vi "TestSurface.vi"() -> ()   [LabVIEW 2024]
uses:
  SDL3/Init/InitFlags--ring.ctl
  <vilib>/picture/picture.llb/imagedata.ctl
  SDL3/Pixels/PixelFormat--enum.ctl
  SDL3/Rect/Rect--cluster.ctl
  SDL3/Init/Init.lvlib
  SDL3/Surface/Surface.lvlib
  SDL3/Rect/Rect.lvlib
  SDL3/Pixels/Pixels.lvlib
  SDL3/Video/Video.lvlib
  SDL3/Video/WindowFlags--ring.ctl
  SDL3/Render/Render.lvlib
  SDL3/Render/TextureAccess-enum.ctl
panel:
  out "new picture 2":picture
  out "color":u32=16711680 format="%06x"
  out "new picture":picture
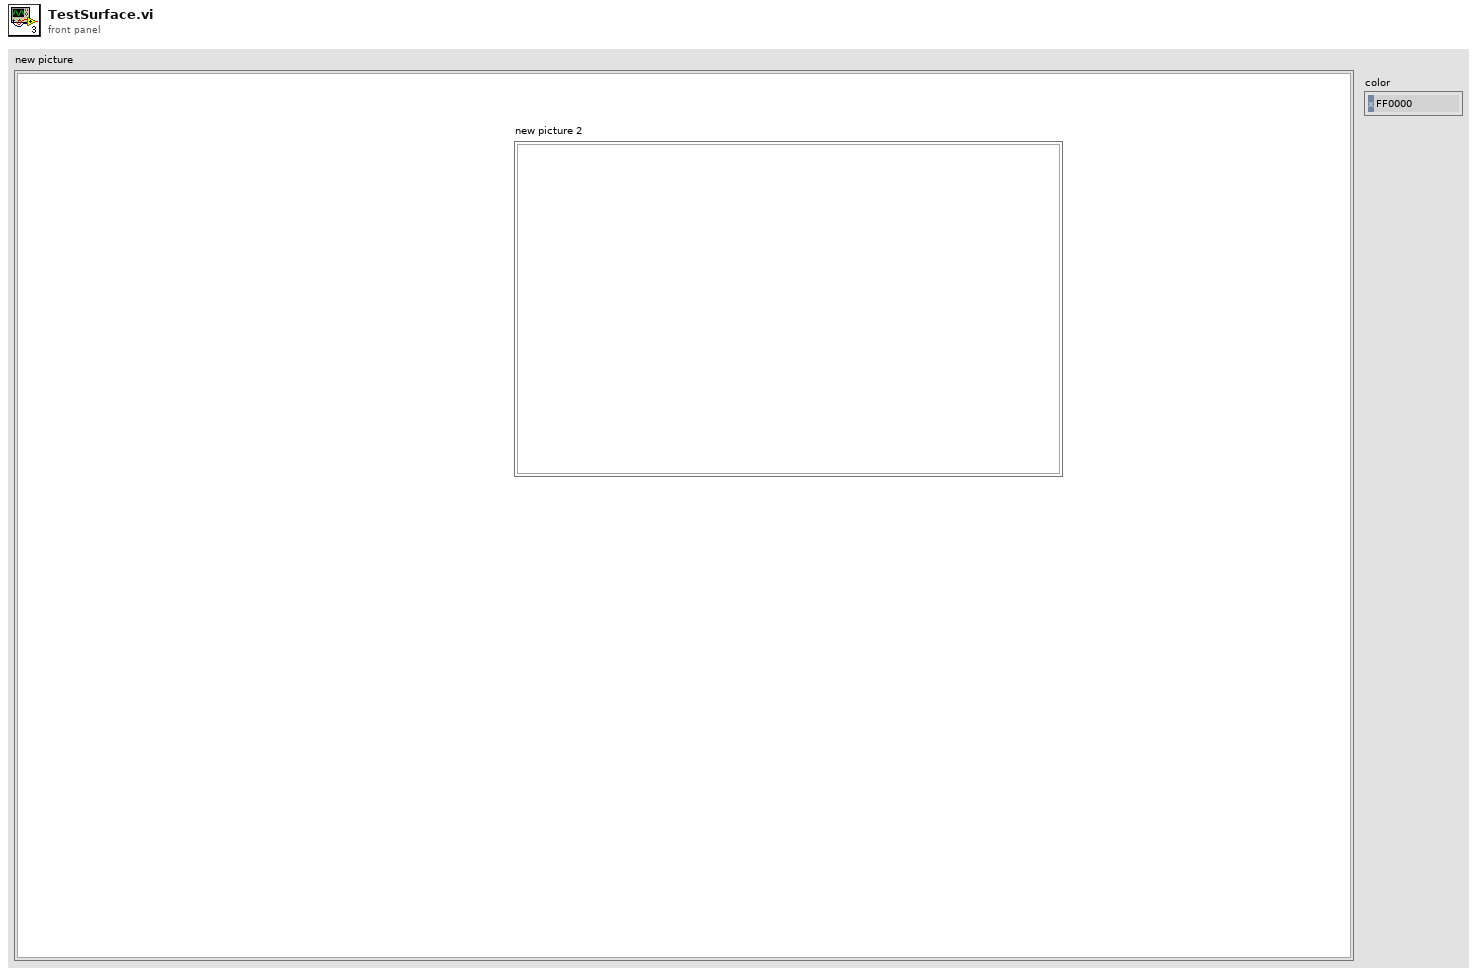
[diagram p1: front panel]
types:
  T1 = typedef "imagedata.ctl" = cluster{"image type":i32, "image depth":i32, "image":u8[], "mask":u8[], "colors":u32[], "Rectangle":cluster{"left":i16, "top":i16, "right":i16, "bottom":i16}}
  T2 = cluster{"left":i16, "top":i16, "right":i16, "bottom":i16}
  T3 = typedef "SDL3.lvlib/Init.lvlib/InitFlags--ring.ctl" = u32
  T4 = typedef "SDL3.lvlib/Render.lvlib/TextureAccess-enum.ctl" = enum32{"SDL_TEXTUREACCESS_STATIC", "SDL_TEXTUREACCESS_STREAMING", "SDL_TEXTUREACCESS_TARGET"}
  T5 = typedef "SDL3.lvlib/Pixels.lvlib/PixelFormat--enum.ctl" = enum32{"SDL_PIXELFORMAT_UNKNOWN", "SDL_PIXELFORMAT_INDEX1LSB", "SDL_PIXELFORMAT_INDEX1MSB", "SDL_PIXELFORMAT_INDEX2LSB", "SDL_PIXELFORMAT_INDEX2MSB", "SDL_PIXELFORMAT_INDEX4LSB", "SDL_PIXELFORMAT_INDEX4MSB", "SDL_PIXELFORMAT_INDEX8", "SDL_PIXELFORMAT_RGB332", "SDL_PIXELFORMAT_XRGB4444", "SDL_PIXELFORMAT_XBGR4444", "SDL_PIXELFORMAT_XRGB1555", "SDL_PIXELFORMAT_XBGR1555", "SDL_PIXELFORMAT_ARGB4444", "SDL_PIXELFORMAT_RGBA4444", "SDL_PIXELFORMAT_ABGR4444", "SDL_PIXELFORMAT_BGRA4444", "SDL_PIXELFORMAT_ARGB1555", "SDL_PIXELFORMAT_RGBA5551", "SDL_PIXELFORMAT_ABGR1555", "SDL_PIXELFORMAT_BGRA5551", "SDL_PIXELFORMAT_RGB565", "SDL_PIXELFORMAT_BGR565", "SDL_PIXELFORMAT_RGB24", "SDL_PIXELFORMAT_BGR24", "SDL_PIXELFORMAT_XRGB8888", "SDL_PIXELFORMAT_RGBX8888", "SDL_PIXELFORMAT_XBGR8888", "SDL_PIXELFORMAT_BGRX8888", "SDL_PIXELFORMAT_ARGB8888", "SDL_PIXELFORMAT_RGBA8888", "SDL_PIXELFORMAT_ABGR8888", "SDL_PIXELFORMAT_BGRA8888", "SDL_PIXELFORMAT_XRGB2101010", "SDL_PIXELFORMAT_XBGR2101010", "SDL_PIXELFORMAT_ARGB2101010", "SDL_PIXELFORMAT_ABGR2101010", "SDL_PIXELFORMAT_RGB48", "SDL_PIXELFORMAT_BGR48", "SDL_PIXELFORMAT_RGBA64", "SDL_PIXELFORMAT_ARGB64", "SDL_PIXELFORMAT_BGRA64", "SDL_PIXELFORMAT_ABGR64", "SDL_PIXELFORMAT_RGB48_FLOAT", "SDL_PIXELFORMAT_BGR48_FLOAT", "SDL_PIXELFORMAT_RGBA64_FLOAT", "SDL_PIXELFORMAT_ARGB64_FLOAT", "SDL_PIXELFORMAT_BGRA64_FLOAT", "SDL_PIXELFORMAT_ABGR64_FLOAT", "SDL_PIXELFORMAT_RGB96_FLOAT", "SDL_PIXELFORMAT_BGR96_FLOAT", "SDL_PIXELFORMAT_RGBA128_FLOAT", "SDL_PIXELFORMAT_ARGB128_FLOAT", "SDL_PIXELFORMAT_BGRA128_FLOAT", "SDL_PIXELFORMAT_ABGR128_FLOAT", "SDL_PIXELFORMAT_YV12", "SDL_PIXELFORMAT_IYUV", "SDL_PIXELFORMAT_YUY2", "SDL_PIXELFORMAT_UYVY", "SDL_PIXELFORMAT_YVYU", "SDL_PIXELFORMAT_NV12", "SDL_PIXELFORMAT_NV21", "SDL_PIXELFORMAT_P010", "SDL_PIXELFORMAT_EXTERNAL_OES"}
  T6 = typedef "SDL3.lvlib/Video.lvlib/WindowFlags--ring.ctl" = u64
  T7 = typedef "SDL3.lvlib/Rect.lvlib/Rect--cluster.ctl" = cluster{"x":i32, "y":i32, "w":i32, "h":i32}
  T8 = typedef "SDL3.lvlib/Surface.lvlib/SurfaceFlags--ring.ctl" = u32
  T9 = cluster{"flag":T8, "format":T5, "w":i32, "h":i32, "pitch":i32}
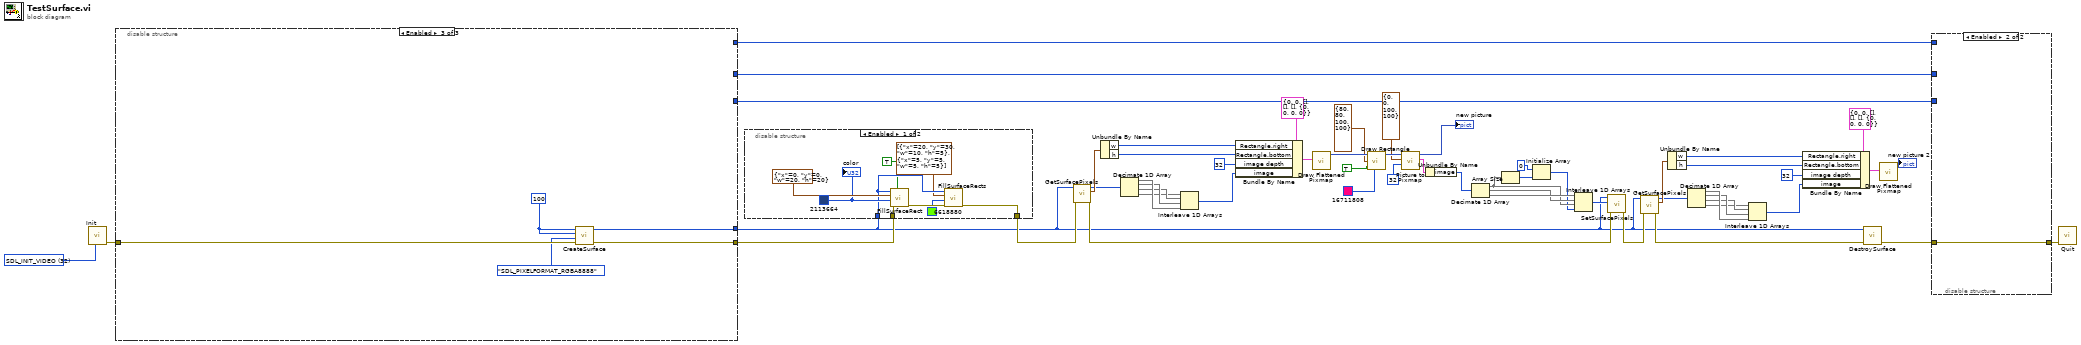
[diagram p0: block diagram]
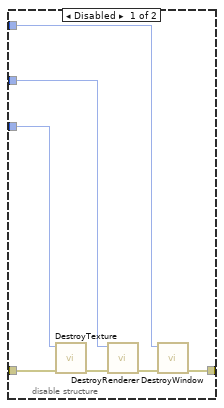
[diagram p2: hidden frame]
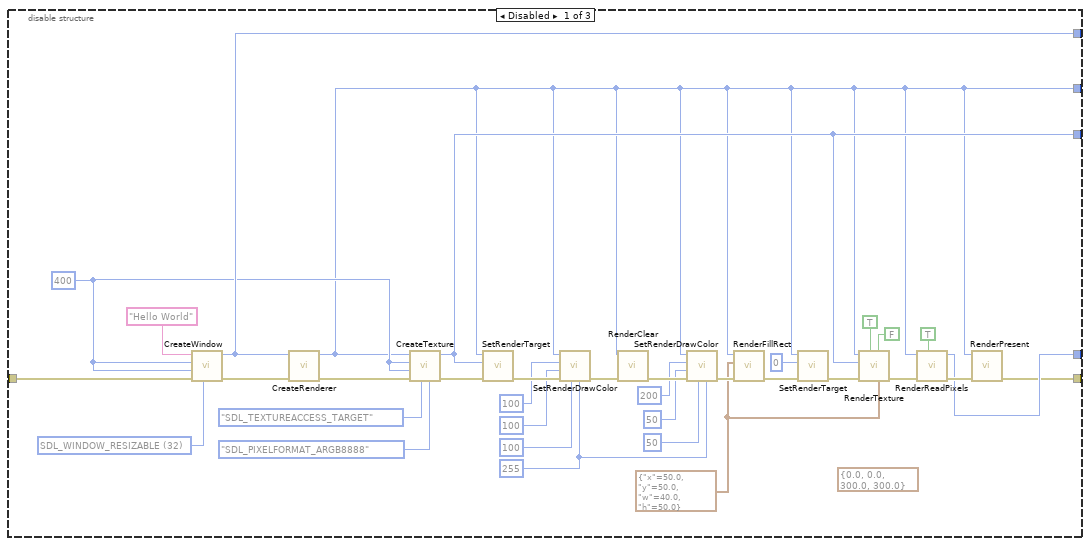
[diagram p3: hidden frame]
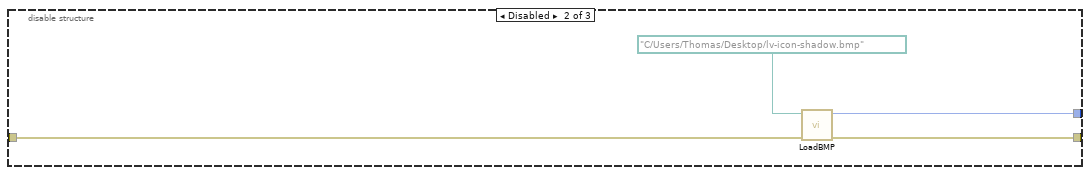
[diagram p4: hidden frame]
diagram:
  w55 = T3 32 items=["NONE"=0, "SDL_INIT_AUDIO"=16, "SDL_INIT_VIDEO"=32, "SDL_INIT_JOYSTICK"=512, "SDL_INIT_HAPTIC"=4096, "SDL_INIT_GAMEPAD"=8192, "SDL_INIT_EVENTS"=16384, "SDL_INIT_SENSOR"=32768, "SDL_INIT_CAMER"=65536] ("InitFlags")
  n1 = call "Init.vi"("InitFlags"=w55) -> ("error out"=w53:errorcluster)  [unwired: 10 in]
  n2 = disable-structure shown="Enabled" {
    disable-tunnel: w53 -> [w84 w93 w98]
    disable-tunnel: [w65 _ _] -> w50
    disable-tunnel: [w64 _ _] -> w49
    disable-tunnel: [w59 w91 w95] -> w1
    disable-tunnel: [w58 w92 w97] -> w47
    disable-tunnel: [w56 _ _] -> w46
    frame Disabled {
      w63 = cluster{"x":sgl, "y":sgl, "w":sgl, "h":sgl} {"x"=50.0, "y"=50.0, "w"=40.0, "h"=50.0} ("rect")
      w68 = u8 255 ("a")
      (unwired) cluster{"x":sgl, "y":sgl, "w":sgl, "h":sgl} {"x"=0.0, "y"=0.0, "w"=300.0, "h"=300.0} ("dstrect")
      w62 = 400 ("h")
      w88 = T6 32 items=["0"=0, "SDL_WINDOW_FULLSCREEN"=1, "SDL_WINDOW_OPENGL"=2, "SDL_WINDOW_OCCLUDED"=4, "SDL_WINDOW_HIDDEN"=8, "SDL_WINDOW_BORDERLESS"=16, "SDL_WINDOW_RESIZABLE"=32, "SDL_WINDOW_MINIMIZED"=64, "SDL_WINDOW_MAXIMIZED"=128, "SDL_WINDOW_MOUSE_GRABBED"=256, "SDL_WINDOW_INPUT_FOCUS"=512, "SDL_WINDOW_MOUSE_FOCUS"=1024, "SDL_WINDOW_EXTERNAL"=2048, "SDL_WINDOW_MODAL"=4096, "SDL_WINDOW_HIGH_PIXEL_DENSITY"=8192, "SDL_WINDOW_MOUSE_CAPTURE"=16384, "SDL_WINDOW_MOUSE_RELATIVE_MODE"=32768, "SDL_WINDOW_ALWAYS_ON_TOP"=65536, "SDL_WINDOW_UTILITY"=131072, "SDL_WINDOW_TOOLTIP"=262144, "SDL_WINDOW_POPUP_MENU"=524288, "SDL_WINDOW_KEYBOARD_GRABBED"=1048576, "SDL_WINDOW_VULKAN"=268435456, "SDL_WINDOW_METAL"=536870912, "SDL_WINDOW_TRANSPARENT"=1073741824, "SDL_WINDOW_NOT_FOCUSABLE"=2147483648] ("flags (0)")
      n3 = call "CreateWindow.vi"("flags (0)"=w88, "No Error"=w84, "h"=w62, "w"=w62, "title"="Hello World") -> ("error out"=w87:errorcluster, "window [SDL_Window *]"=w64:i64)  [unwired: 5 in]
      n4 = call "CreateRenderer.vi"("No Error"=w87, "window [SDL_Window *]"=w64) -> ("error out"=w86:errorcluster, "renderer [SDL_Renderer *]"=w56:i64)  [unwired: 8 in]
      n5 = call "CreateTexture.vi"("pixel_format"=PixelFormat--enum."SDL_PIXELFORMAT_ARGB8888", "texture_access"=TextureAccess-enum."SDL_TEXTUREACCESS_TARGET", "No Error"=w86, "h"=w62, "w"=w62, "renderer [SDL_Renderer *]"=w56) -> ("error out"=w66:errorcluster, "texture [SDL_Texture *]"=w65:i64)  [unwired: 4 in]
      n6 = call "SetRenderTarget.vi"("No Error"=w66, "texture [SDL_Texture *]"=w65, "renderer [SDL_Renderer *]"=w56) -> ("error out"=w81:errorcluster)  [unwired: 8 in]
      n7 = call "SetRenderDrawColor.vi"("a"=w68, "b"=u8 100, "No Error"=w81, "g"=u8 100, "r"=u8 100, "renderer [SDL_Renderer *]"=w56) -> ("error out"=w79:errorcluster)  [unwired: 5 in]
      n8 = call "RenderClear.vi"("No Error"=w79, "renderer [SDL_Renderer *]"=w56) -> ("error out"=w80:errorcluster)  [unwired: 9 in]
      n9 = call "SetRenderDrawColor.vi"("a"=w68, "b"=u8 50, "No Error"=w80, "g"=u8 50, "r"=u8 200, "renderer [SDL_Renderer *]"=w56) -> ("error out"=w72:errorcluster)  [unwired: 5 in]
      n10 = call "RenderFillRect.vi"("No Error"=w72, "rect"=w63, "renderer [SDL_Renderer *]"=w56) -> ("error out"=w67:errorcluster)  [unwired: 8 in]
      n11 = call "SetRenderTarget.vi"("No Error"=w67, "texture [SDL_Texture *]"=i64 0, "renderer [SDL_Renderer *]"=w56) -> ("error out"=w82:errorcluster)  [unwired: 8 in]
      n12 = call "RenderTexture.vi"("dstrect"=w63, "Entire Rendering Target (F)"=FALSE, "Entire Texture (F)"=TRUE, "No Error"=w82, "texture [SDL_Texture *]"=w65, "renderer [SDL_Renderer *]"=w56) -> ("error out"=w61:errorcluster)  [unwired: 5 in]
      n13 = call "RenderReadPixels.vi"("Entire Viewport? (F)"=TRUE, "No Error"=w61, "renderer [SDL_Renderer *]"=w56) -> ("error out"=w60:errorcluster, "surface [SDL_Surface *]"=w59:i64)  [unwired: 7 in]
      n14 = call "RenderPresent.vi"("No Error"=w60, "renderer [SDL_Renderer *]"=w56) -> ("error out"=w58:errorcluster)  [unwired: 9 in]
    }
    frame Disabled {
      n15 = call "LoadBMP.vi"("No Error"=w93, "file"=path "C:/Users/Thomas/Desktop/lv-icon-shadow.bmp") -> ("error out"=w92:errorcluster, "surface [SDL_Surface *]"=w91:i64)  [unwired: 8 in]
    }
    frame Enabled {
      w96 = 100 ("width")
      n16 = call "CreateSurface.vi"("No Error"=w98, "format"=PixelFormat--enum."SDL_PIXELFORMAT_RGBA8888", "height"=w96, "width"=w96) -> ("error out"=w97:errorcluster, "surface [SDL_Surface *]"=w95:i64)  [unwired: 6 in]
    }
  }
  n17 = disable-structure shown="Enabled" {
    disable-tunnel: w47 -> [w107 w108]
    disable-tunnel: [w103 w108] -> w54
    disable-tunnel: w1 -> [w101 _]
    frame Enabled {
      w105 = u32 2113664 ("color")
      n18 = call "FillSurfaceRect.vi"("Entire Surface (F)"=TRUE, "No Error"=w107, "color"=w105, "rect"=T7 {"x"=0, "y"=0, "w"=20, "h"=20}, "dst [SDL_Surface *]"=w101) -> ("error out"=w104:errorcluster)  [unwired: 6 in]
      n19 = call "FillSurfaceRects.vi"("No Error"=w104, "color"=u32 6618880, "rects"=T7[] [{"x"=20, "y"=30, "w"=10, "h"=5}, {"x"=5, "y"=5, "w"=5, "h"=5}], "dst [SDL_Surface *]"=w101) -> ("error out"=w103:errorcluster)  [unwired: 7 in]
      "color" <- w105
    }
    frame Disabled {
    }
  }
  n20 = call "GetSurfacePixels.vi"("No Error"=w54, "surface [SDL_Surface *]"=w1) -> ("error out"=w17:errorcluster, "Surface Info"=w48:T9, "Pixels"=w36:u8[])  [unwired: 7 in]
  n21 = Unbundle By Name(w48) -> ("w"=w42:i32, "h"=w41:i32)
  n22 = Decimate 1D Array(w36) -> (w40:u8[], w39:u8[], w38:u8[], w37:u8[])
  n23 = Interleave 1D Arrays(w37, w38, w39, w40) -> (w35:u8[])
  n24 = Bundle By Name(cluster=T1 {"image type"=0, "image depth"=0, "image"=[], "mask"=[], "colors"=[], "Rectangle"={"left"=0, "top"=0, "right"=0, "bottom"=0}} ("image data"), "Rectangle.right"=w42, "Rectangle.bottom"=w41, "image depth"=32, "image"=w35) -> (w44:T1)
  n25 = call <vilib>:"Draw Flattened Pixmap.vi"("image data"=w44) -> ("new picture"=w34:picture)  [unwired: 8 in]
  n26 = call <vilib>:"Draw Rectangle.vi"("picture"=w34, "rect"=T2 {"left"=80, "top"=80, "right"=100, "bottom"=100}, "fill?(F)"=TRUE, "color(black)"=u32 16711808) -> ("new picture"=w30:picture)  [unwired: 5 in]
  n27 = call <vilib>:"Picture to Pixmap.vi"("depth"=32, "rect"=T2 {"left"=0, "top"=0, "right"=100, "bottom"=100}, "picture"=w30) -> ("image data"=w26:T1, "new picture"=→"new picture":picture)  [unwired: 7 in]
  n28 = Unbundle By Name(w26) -> ("image"=w25:u8[])
  n29 = Decimate 1D Array(w25) -> (w20:u8[], w21:u8[], w22:u8[])
  n30 = Array Size(array=w20) -> (size(s)=w24:i32)
  n31 = Initialize Array(u8 0 ("element"), w24) -> (w19:u8[])
  n32 = Interleave 1D Arrays(w22, w21, w20, w19) -> (w18:u8[])
  n33 = call "SetSurfacePixels.vi"("No Error"=w17, "Pixels"=w18, "surface [SDL_Surface *]"=w1) -> ("error out"=w4:errorcluster)  [unwired: 8 in]
  n34 = call "GetSurfacePixels.vi"("No Error"=w4, "surface [SDL_Surface *]"=w1) -> ("error out"=w3:errorcluster, "Surface Info"=w16:T9, "Pixels"=w6:u8[])  [unwired: 7 in]
  n35 = Unbundle By Name(w16) -> ("w"=w12:i32, "h"=w11:i32)
  n36 = Decimate 1D Array(w6) -> (w10:u8[], w9:u8[], w8:u8[], w7:u8[])
  n37 = Interleave 1D Arrays(w7, w8, w9, w10) -> (w5:u8[])
  n38 = Bundle By Name(cluster=T1 {"image type"=0, "image depth"=0, "image"=[], "mask"=[], "colors"=[], "Rectangle"={"left"=0, "top"=0, "right"=0, "bottom"=0}} ("image data"), "Rectangle.right"=w12, "Rectangle.bottom"=w11, "image depth"=32, "image"=w5) -> (w14:T1)
  n39 = call "DestroySurface.vi"("No Error"=w3, "surface [SDL_Surface *]"=w1) -> ("error out"=w52:errorcluster)  [unwired: 9 in]
  n40 = call <vilib>:"Draw Flattened Pixmap.vi"("image data"=w14) -> ("new picture"=→"new picture 2":picture)  [unwired: 8 in]
  n41 = disable-structure shown="Enabled" {
    disable-tunnel: w52 -> [w113 w116]
    disable-tunnel: [w112 w116] -> w51
    disable-tunnel: w50 -> [w111 _]
    disable-tunnel: w49 -> [w110 _]
    disable-tunnel: w46 -> [w109 _]
    frame Disabled {
      n42 = call "DestroyTexture.vi"("No Error"=w113, "texture [SDL_Texture *]"=w111) -> ("error out"=w114:errorcluster)  [unwired: 9 in]
      n43 = call "DestroyRenderer.vi"("No Error"=w114, "renderer [SDL_Renderer *]"=w109) -> ("error out"=w115:errorcluster)  [unwired: 9 in]
      n44 = call "DestroyWindow.vi"("No Error"=w115, "window [SDL_Window*]"=w110) -> ("error out"=w112:errorcluster)  [unwired: 9 in]
    }
    frame Enabled {
    }
  }
  n45 = call "Quit.vi"("No Error"=w51) -> ()  [unwired: 10 in, 1 out]
